vi "Diagrams get.vi"(0 "GObjects[]":refnum<vi>[](array[refnum]), 11 "error in (no error)":errorcluster) -> (4 "Diagrams[]":refnum<vi>[](array[refnum]), 15 "error out":errorcluster)   [LabVIEW 2012, in "ColourUpStructures.lvlib"]
doc: "If <b>GObjects[]</b> is FlatSequence or Structure then extract and return its <b>Diagrams</b>"
uses:
  ColourUpStructures.lvlib
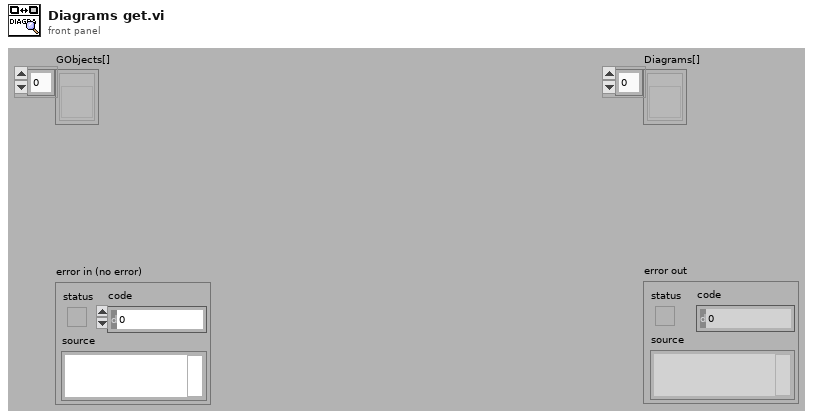
[diagram p1: front panel]
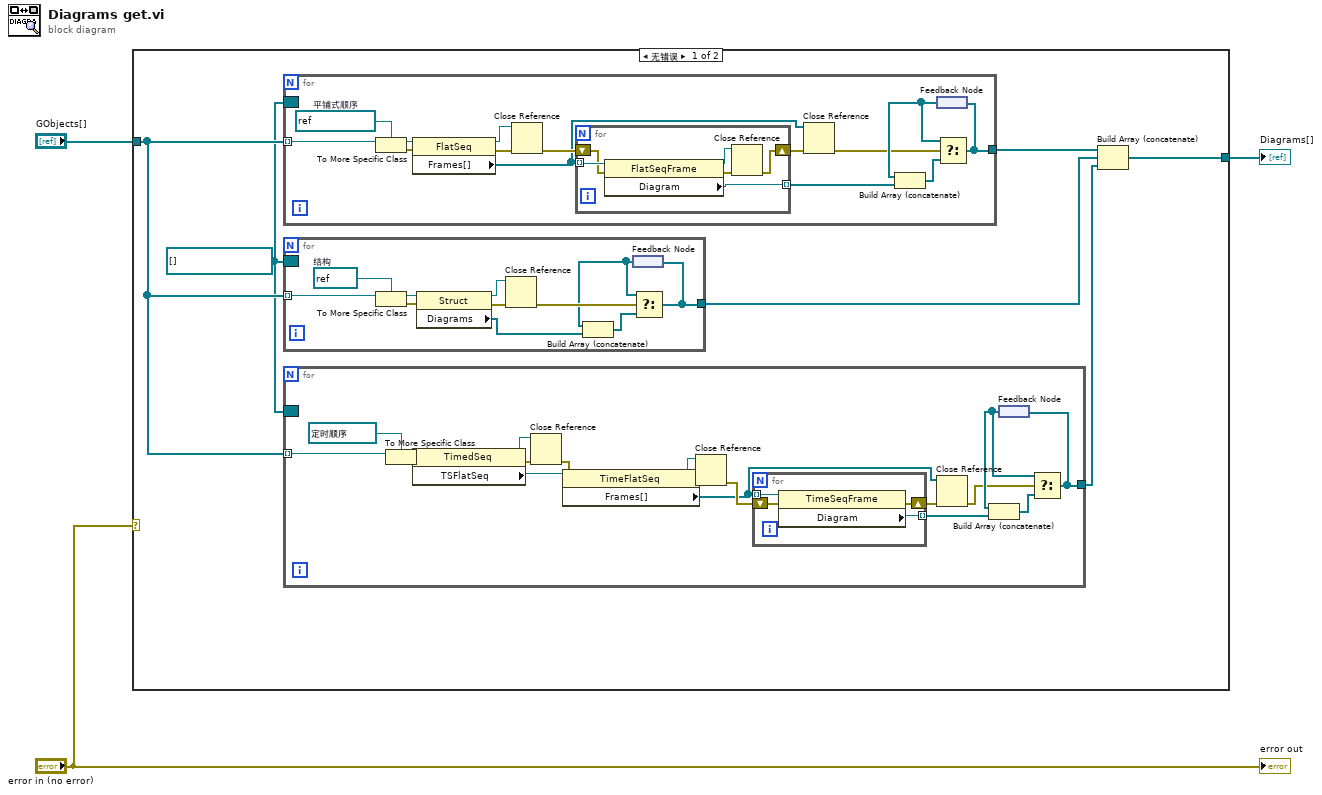
[diagram p0: block diagram]
diagram:
  n1 = case shown="无错误" "error in (no error)" {
    tunnel: "GObjects[]" -> [w6 _]
    tunnel: [w7 _] -> w2
    frame No Error {
      w5 = refnum<vi>[] []
      n2 = for {
        tunnel: w6 -> [w56] mode=indexing
        border: w5 -> [_]
        tunnel: [w46] -> w9
        w55 = refnum<vi> refnum  # 平铺式顺序
        n3 = To More Specific Class(target class=w55, reference=w56) -> (specific class reference=w54:refnum<vi>, error out=w53:errorcluster)  [unwired: 1 in]
        n4 = property class="FlatSeq"(reference=w54, error in=w53) -> (reference out=w52:refnum<vi>, error out=w51:errorcluster, "Frames[]"=w43:refnum<vi>[])
        n5 = Close Reference(reference=w52, error in (no error)=w51) -> (error out=w50:errorcluster)
        n6 = for {
          tunnel: w43 -> [w62] mode=indexing
          shift-right: [w58] -> w45
          shift-left: w50 -> [w59]
          tunnel: [w57] -> w49 mode=indexing
          n7 = property class="FlatSeqFrame"(reference=w62, error in=w59) -> (reference out=w60:refnum<vi>, error out=w61:errorcluster, "Diagram"=w57:refnum<vi>)
          n8 = Close Reference(reference=w60, error in (no error)=w61) -> (error out=w58:errorcluster)
        }
        n9 = Close Reference(reference=w43, error in (no error)=w45) -> (error out=w44:errorcluster)
        n10 = feedback #1() -> (w47:refnum<vi>[])
        n11 = Build Array (concatenate)(w47, w49) -> (w48:refnum<vi>[])
        n12 = Select(t=w47, s=w44, f=w48) -> (s? t:f=w46:refnum<vi>[])
        n13 = feedback-in #1(w46) -> ()
      }
      n14 = for {
        tunnel: w6 -> [w42] mode=indexing
        border: w5 -> [_]
        tunnel: [w32] -> w8
        w41 = refnum<vi> refnum  # 结构
        n15 = To More Specific Class(target class=w41, reference=w42) -> (specific class reference=w40:refnum<vi>, error out=w39:errorcluster)  [unwired: 1 in]
        n16 = property class="Struct"(reference=w40, error in=w39) -> (reference out=w37:refnum<vi>, error out=w38:errorcluster, "Diagrams"=w35:refnum<vi>[])
        n17 = Close Reference(reference=w37, error in (no error)=w38) -> (error out=w36:errorcluster)
        n18 = feedback #2() -> (w33:refnum<vi>[])
        n19 = Build Array (concatenate)(w33, w35) -> (w34:refnum<vi>[])
        n20 = Select(t=w33, s=w36, f=w34) -> (s? t:f=w32:refnum<vi>[])
        n21 = feedback-in #2(w32) -> ()
      }
      n22 = for {
        tunnel: w6 -> [w27] mode=indexing
        border: w5 -> [_]
        tunnel: [w10] -> w4
        n23 = To More Specific Class(target class=refnum<vi> refnum ("owner refnum"), reference=w27) -> (specific class reference=w25:refnum<vi>, error out=w24:errorcluster)  [unwired: 1 in]
        n24 = property class="TimedSeq"(reference=w25, error in=w24) -> (reference out=w20:refnum<vi>, error out=w12:errorcluster, "TSFlatSeq"=w23:refnum<vi>)
        n25 = Close Reference(reference=w20, error in (no error)=w12) -> (error out=w11:errorcluster)
        n26 = property class="TimeFlatSeq"(reference=w23, error in=w11) -> (reference out=w18:refnum<vi>, error out=w19:errorcluster, "Frames[]"=w15:refnum<vi>[])
        n27 = Close Reference(reference=w18, error in (no error)=w19) -> (error out=w17:errorcluster)
        n28 = for {
          tunnel: w15 -> [w31] mode=indexing
          shift-right: [w29] -> w16
          shift-left: w17 -> [w30]
          tunnel: [w28] -> w14 mode=indexing
          n29 = property class="TimeSeqFrame"(reference=w31, error in=w30) -> (error out=w29:errorcluster, "Diagram"=w28:refnum<vi>)  [unwired: 1 out]
        }
        n30 = Close Reference(reference=w15, error in (no error)=w16) -> (error out=w21:errorcluster)
        n31 = feedback #3() -> (w22:refnum<vi>[])
        n32 = Build Array (concatenate)(w22, w14) -> (w13:refnum<vi>[])
        n33 = Select(t=w22, s=w21, f=w13) -> (s? t:f=w10:refnum<vi>[])
        n34 = feedback-in #3(w10) -> ()
      }
      n35 = Build Array (concatenate)(w9, w8, w4) -> (w7:refnum<vi>[])
    }
    frame Error {
    }
  }
  "Diagrams[]" <- w2
  "error out" <- "error in (no error)"
